vi "ServerStatusMessage.vi"(11 "Error Status":string) -> (3 "Message out":string)   [LabVIEW 2011]
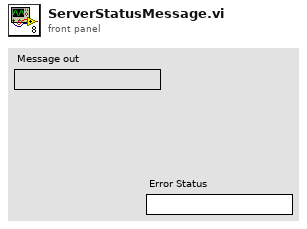
[diagram p1: front panel]
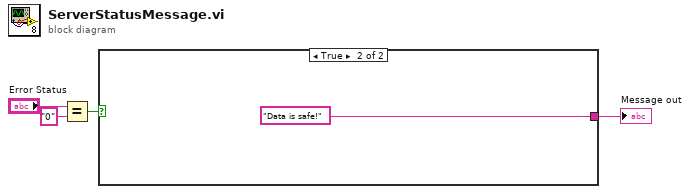
[diagram p0: block diagram]
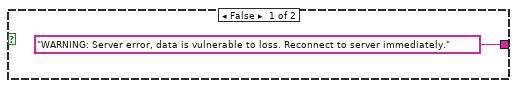
[diagram p2: hidden frame]
diagram:
  n1 = Equal?(x="Error Status", y="0") -> (x = y?=w2:bool)
  n2 = case shown="True" w2 {
    tunnel: ["WARNING: Server error, data is vulnerable to loss. Reconnect to server immediately." "Data is safe!"] -> w1
    frame False {
    }
    frame True {
    }
  }
  "Message out" <- w1
